vi "ShoulderNetworkingGlobal.vi"() -> ()   [LabVIEW 2023]
panel:
  out "LiftFowardLimit":bool
  out "LiftFowardLimitL":bool
  out "LiftFowardLimitR":bool
  out "OnTarget":bool
  in  "LiftSensorPosition":dbl
  in  "LiftDemand":dbl
  in  "MotorOutput":dbl
  # "#TODO Combine Shoulder globals into a single global VI"
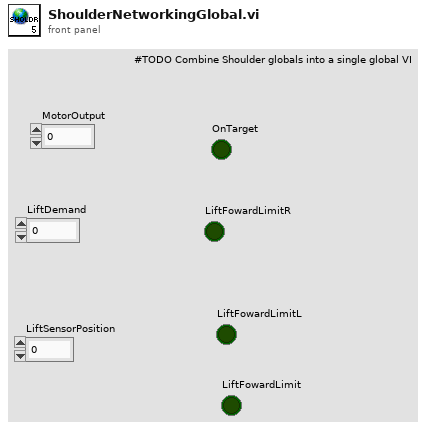
[diagram p1: front panel]
diagram:
